vi "Сумматор.vi"(2 "i-1":bool, 3 "B":bool, 4 "A":bool) -> (0 "Ci":bool, 1 "Si":bool)   [LabVIEW 2017]
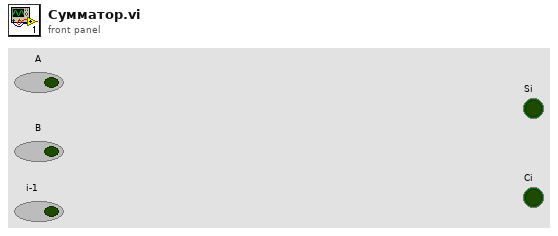
[diagram p1: front panel]
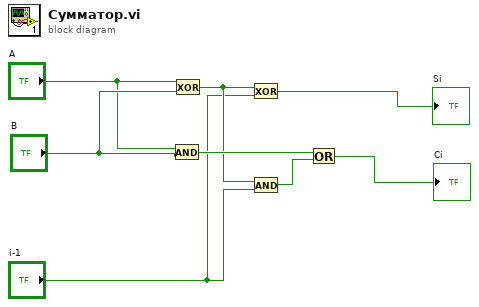
[diagram p0: block diagram]
diagram:
  n1 = And(x="A", y="B") -> (x .and. y?=w6:bool)
  n2 = Exclusive Or(1:"B", 2:"A") -> (0:w2:bool)
  n3 = Exclusive Or(1:"i-1", 2:w2) -> (0:→"Si":bool)
  n4 = And(x=w2, y="i-1") -> (x .and. y?=w5:bool)
  n5 = Or(x=w6, y=w5) -> (x .or. y?=→"Ci":bool)
